vi "testExtractElementName.vi"(8 "error in (no error)":errorcluster) -> (0 "error out":errorcluster)   [LabVIEW 2018]
uses:
  SALTypeGenerator/Topic/Topic.lvclass
  SALTypeGenerator/Topic/Topic.lvclass/Topic.ctl
  <vilib>/addons/_JKI Toolkits/Caraya/classes/Assert/Assert Equal Value_Variant.vi
  <vilib>/addons/_JKI Toolkits/Caraya/classes/Test/Test.lvclass
  <vilib>/addons/_JKI Toolkits/Caraya/classes/Assert/Assert.lvclass
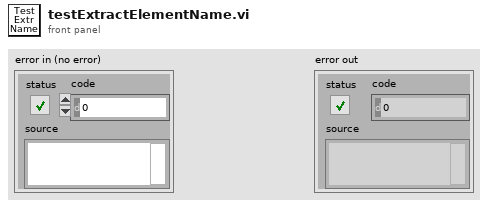
[diagram p1: front panel]
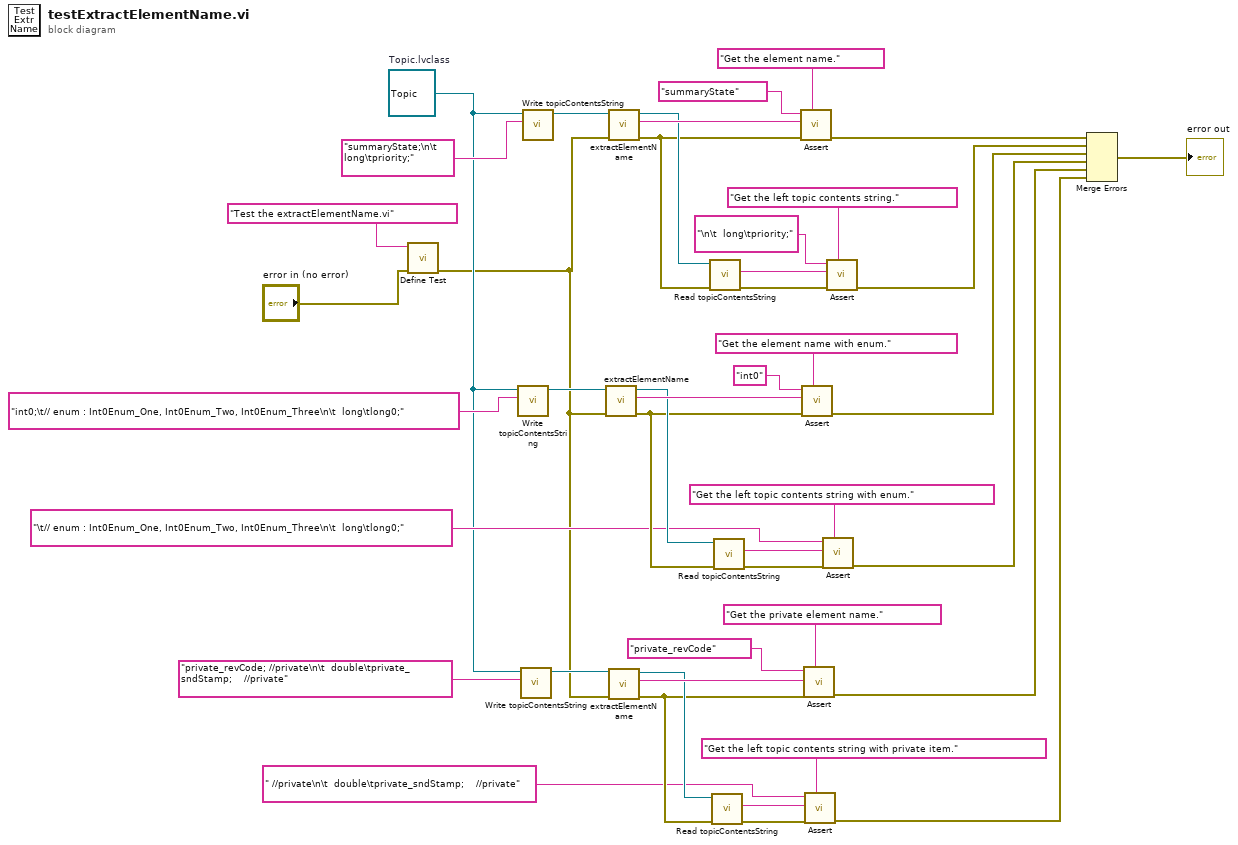
[diagram p0: block diagram]
diagram:
  w15 = refnum<class "Topic.lvclass"> refnum  # Topic.lvclass
  n1 = call <vilib>:"Define Test.vi"("error in (no error)"="error in (no error)", "Label (VI Title)"="Test the extractElementName.vi") -> ("error out"=w12:errorcluster)  [unwired: 9 in]
  n2 = call "Write topicContentsString.vi"("topicContentsString"="int0;\t// enum : Int0Enum_One, Int0Enum_Two, Int0Enum_Three\n\t  long\tlong0;", "Topic in"=w15) -> ("Topic out"=w27:refnum<class "Topic.lvclass">)  [unwired: 9 in]
  n3 = call "Write topicContentsString.vi"("topicContentsString"="private_revCode; //private\n\t  double\tprivate_sndStamp;    //private", "Topic in"=w15) -> ("Topic out"=w13:refnum<class "Topic.lvclass">)  [unwired: 9 in]
  n4 = call "Write topicContentsString.vi"("topicContentsString"="summaryState;\n\t  long\tpriority;", "Topic in"=w15) -> ("Topic out"=w41:refnum<class "Topic.lvclass">)  [unwired: 9 in]
  n5 = call "extractElementName.vi"("error in (no error)"=w12, "Topic in"=w27) -> ("error out"=w24:errorcluster, "elementName"=w26:string, "Topic out"=w25:refnum<class "Topic.lvclass">)  [unwired: 7 in]
  n6 = call "extractElementName.vi"("error in (no error)"=w12, "Topic in"=w41) -> ("error out"=w36:errorcluster, "elementName"=w40:string, "Topic out"=w37:refnum<class "Topic.lvclass">)  [unwired: 7 in]
  n7 = call "extractElementName.vi"("error in (no error)"=w12, "Topic in"=w13) -> ("error out"=w6:errorcluster, "elementName"=w11:string, "Topic out"=w7:refnum<class "Topic.lvclass">)  [unwired: 7 in]
  n8 = call "Read topicContentsString.vi"("error in (no error)"=w36, "Topic in"=w37) -> ("error out"=w35:errorcluster, "topicContentsString"=w34:string)  [unwired: 7 in, 1 out]
  n9 = call "Read topicContentsString.vi"("error in (no error)"=w6, "Topic in"=w7) -> ("error out"=w5:errorcluster, "topicContentsString"=w4:string)  [unwired: 7 in, 1 out]
  n10 = call "Read topicContentsString.vi"("error in (no error)"=w24, "Topic in"=w25) -> ("error out"=w23:errorcluster, "topicContentsString"=w22:string)  [unwired: 7 in, 1 out]
  n11 = call-poly <vilib>:"Assert.vi"("Label"="Get the element name.", "error in (no error)"=w36, "Y"=w40, "X"="summaryState") -> ("error out"=w32:errorcluster)  [unwired: 7 in]
  n12 = call-poly <vilib>:"Assert.vi"("Label"="Get the element name with enum.", "error in (no error)"=w24, "Y"=w26, "X"="int0") -> ("error out"=w18:errorcluster)  [unwired: 7 in]
  n13 = call-poly <vilib>:"Assert.vi"("Label"="Get the private element name.", "error in (no error)"=w6, "Y"=w11, "X"="private_revCode") -> ("error out"=w8:errorcluster)  [unwired: 7 in]
  n14 = call-poly <vilib>:"Assert.vi"("Label"="Get the left topic contents string with private item.", "error in (no error)"=w5, "Y"=w4, "X"=" //private\n\t  double\tprivate_sndStamp;    //private") -> ("error out"=w2:errorcluster)  [unwired: 7 in]
  n15 = call-poly <vilib>:"Assert.vi"("Label"="Get the left topic contents string with enum.", "error in (no error)"=w23, "Y"=w22, "X"="\t// enum : Int0Enum_One, Int0Enum_Two, Int0Enum_Three\n\t  long\tlong0;") -> ("error out"=w17:errorcluster)  [unwired: 7 in]
  n16 = call-poly <vilib>:"Assert.vi"("Label"="Get the left topic contents string.", "error in (no error)"=w35, "Y"=w34, "X"="\n\t  long\tpriority;") -> ("error out"=w31:errorcluster)  [unwired: 7 in]
  n17 = Merge Errors(w32, w31, w18, w17, w8, w2) -> (→"error out":errorcluster)
